vi "plus_minus_plus.vi"(1 "4":dbl, 2 "3":dbl, 3 "2":dbl, 4 "1":dbl=1.0) -> (0 "숫자형 출력":dbl)   [LabVIEW 2018]
doc: "사칙연산을 할것 같지만 안합니다."
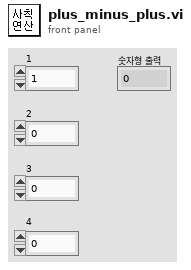
[diagram p1: front panel]
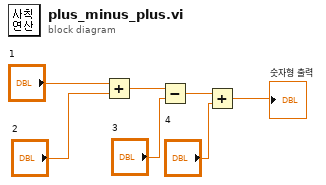
[diagram p0: block diagram]
diagram:
  n1 = Add ("더하기")(x="1", y="2") -> (x+y=w3:dbl)
  n2 = Subtract ("빼기")(x=w3, y="3") -> (x-y=w6:dbl)
  n3 = Add ("더하기")(x=w6, y="4") -> (x+y=→"숫자형 출력":dbl)
